vi "niDTS WLAN INSTR TX Fetch DSSS Results.vi"(8 "error in (no error)":errorcluster, 10 "ActiveResultsSpace":u8=1, 11 "niDTS WLAN INSTR TX in":refnum<class "niDTS WLAN INSTR TX.lvclass">) -> (0 "error out":errorcluster, 2 "DSSS Results":T1 {"OBW"."Stop Frequency (Hz)" format="%#_4p"; "OBW"."Start Frequency (Hz)" format="%#_4p"; "OBW"."OBW (Hz)" format="%#_4p"}, 3 "niDTS WLAN INSTR TX out":refnum<class "niDTS WLAN INSTR TX.lvclass">)   [LabVIEW 2015, in "niDTS WLAN.lvlib" / "niDTS WLAN INSTR TX.lvclass"]
uses:
  niDTS WLAN INSTR TX.lvclass
  Tests/Tx Test/Includes/niDTS WLAN Tx Test INC DSSS Results.ctl
  Tests/Tx Test/Includes/niDTS WLAN Tx Test INC DSSS MOD EVM Results.ctl
  Tests/DSSS Tx Test/Includes/Results/niDTS WLAN DSSS Tx RES EVM ALL.ctl
  Tests/DSSS Tx Test/Includes/Results/niDTS WLAN DSSS Tx RES EVM RMS.ctl
  Tests/Tx Test/Includes/niDTS WLAN Tx Test INC TXP Results.ctl
  Tests/Tx Test/Includes/niDTS WLAN Tx Test INC TXP Result SINGLE.ctl
  Tests/Tx Test/Includes/niDTS WLAN Tx Test INC OBW Results.ctl
  Results/niDTS WLAN INSTR TX INC SEM Results.ctl
  Results/niDTS WLAN INSTR TX INC SEM FSEGemts Results.ctl
  Tests/Tx Test/Includes/Results/niDTS Tx RES INC SEM FSEGemts.ctl
  Results/niDTS WLAN INSTR TX INC SEM MARGin Results.ctl
  Tests/Tx Test/Includes/Results/niDTS Tx RES INC SEM Margin.ctl
  Tests/Tx Test/Includes/niDTS WLAN Tx Test INC DSSS MOD Impairments Results.ctl
  Tests/DSSS Tx Test/Includes/Results/niDTS WLAN DSSS Tx Impairmentsctl.ctl
  Tests/DSSS Tx Test/Includes/Results/niDTS WLAN DSSS Tx PowerRamp.ctl
  niDTS WLAN.lvlib
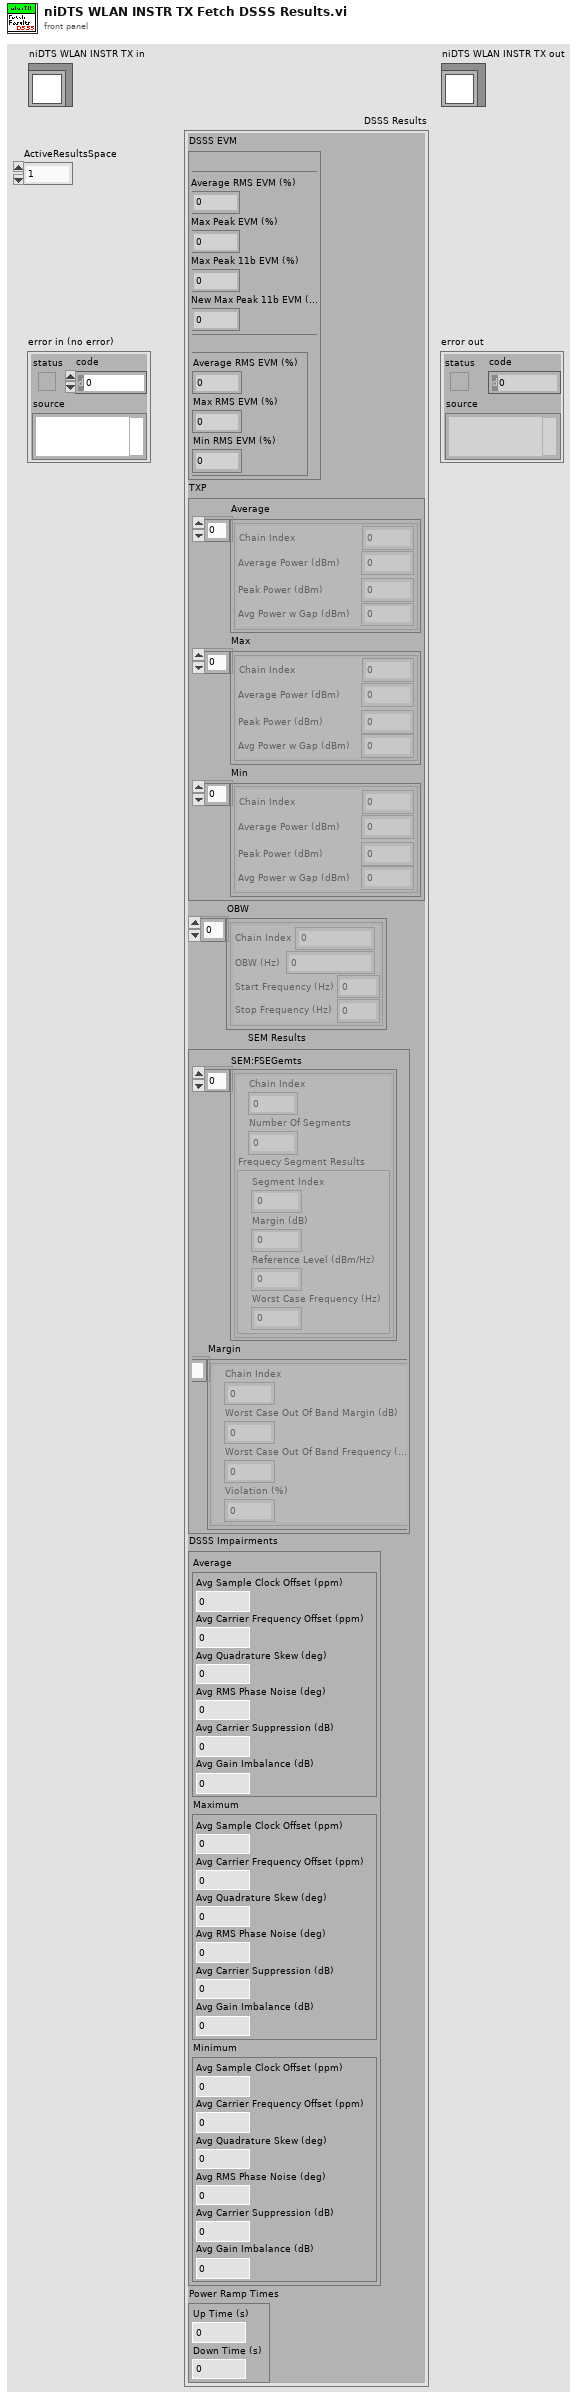
[diagram p1: front panel]
types:
  T1 = typedef "niDTS WLAN.lvlib/niDTS WLAN Tx Test INC DSSS Results.ctl" = cluster{"DSSS EVM":T2, "TXP":T5, "OBW":T7[], "SEM Results":T8, "DSSS Impairments":T13, "Power Ramp Times":T15}
  T2 = typedef "niDTS WLAN.lvlib/niDTS WLAN Tx Test INC DSSS MOD EVM Results.ctl" = cluster{"All":T3, "RMS":T4}
  T3 = typedef "niDTS WLAN.lvlib/niDTS WLAN DSSS Tx RES EVM ALL.ctl" = cluster{"Average RMS EVM (%)":dbl, "Max Peak EVM (%)":dbl, "Max Peak 11b EVM (%)":dbl, "New Max Peak 11b EVM (%)":dbl}
  T4 = typedef "niDTS WLAN.lvlib/niDTS WLAN DSSS Tx RES EVM RMS.ctl" = cluster{"Average RMS EVM (%)":dbl, "Max RMS EVM (%)":dbl, "Min RMS EVM (%)":dbl}
  T5 = typedef "niDTS WLAN.lvlib/niDTS WLAN Tx Test INC TXP Results.ctl" = cluster{"Average":T6[], "Max":T6[], "Min":T6[]}
  T6 = typedef "niDTS WLAN.lvlib/niDTS WLAN Tx Test INC TXP Result SINGLE.ctl" = cluster{"Chain Index":dbl, "Average Power (dBm)":dbl, "Peak Power (dBm)":dbl, "Avg Power w Gap (dBm)":dbl}
  T7 = typedef "niDTS WLAN.lvlib/niDTS WLAN Tx Test INC OBW Results.ctl" = cluster{"Chain Index":dbl, "OBW (Hz)":dbl, "Start Frequency (Hz)":dbl, "Stop Frequency (Hz)":dbl}
  T8 = typedef "niDTS WLAN.lvlib/niDTS WLAN INSTR TX.lvclass/niDTS WLAN INSTR TX INC SEM Results.ctl" = cluster{"SEM:FSEGemts":T9, "Margin":T11}
  T9 = typedef "niDTS WLAN.lvlib/niDTS WLAN INSTR TX.lvclass/niDTS WLAN INSTR TX INC SEM FSEGemts Results.ctl" = T10[]
  T10 = typedef "niDTS WLAN.lvlib/niDTS Tx RES INC SEM FSEGemts.ctl" = cluster{"Chain Index":i32, "Number Of Segments":i32, "Frequecy Segment Results":cluster{"Segment Index":i32, "Margin (dB)":dbl, "Reference Level (dBm/Hz)":dbl, "Worst Case Frequency (Hz)":dbl}}
  T11 = typedef "niDTS WLAN.lvlib/niDTS WLAN INSTR TX.lvclass/niDTS WLAN INSTR TX INC SEM MARGin Results.ctl" = T12[]
  T12 = typedef "niDTS WLAN.lvlib/niDTS Tx RES INC SEM Margin.ctl" = cluster{"Chain Index":i32, "Worst Case Out Of Band Margin (dB)":dbl, "Worst Case Out Of Band Frequency (Hz)":dbl, "Violation (%)":dbl}
  T13 = typedef "niDTS WLAN.lvlib/niDTS WLAN Tx Test INC DSSS MOD Impairments Results.ctl" = cluster{"Average":T14, "Maximum":T14, "Minimum":T14}
  T14 = typedef "niDTS WLAN.lvlib/niDTS WLAN DSSS Tx Impairmentsctl.ctl" = cluster{"Avg Sample Clock Offset (ppm)":dbl, "Avg Carrier Frequency Offset (ppm)":dbl, "Avg Quadrature Skew (deg)":dbl, "Avg RMS Phase Noise (deg)":dbl, "Avg Carrier Suppression (dB)":dbl, "Avg Gain Imbalance (dB)":dbl}
  T15 = typedef "niDTS WLAN.lvlib/niDTS WLAN DSSS Tx PowerRamp.ctl" = cluster{"Up Time (s)":dbl, "Down Time (s)":dbl}
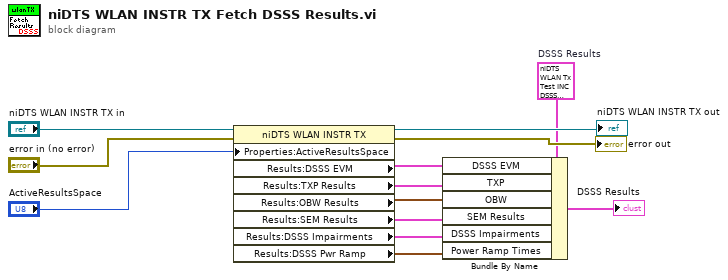
[diagram p0: block diagram]
diagram:
  w8 = T1 {"DSSS EVM"={"All"={"Average RMS EVM (%)"=0.0, "Max Peak EVM (%)"=0.0, "Max Peak 11b EVM (%)"=0.0, "New Max Peak 11b EVM (%)"=0.0}, "RMS"={"Average RMS EVM (%)"=0.0, "Max RMS EVM (%)"=0.0, "Min RMS EVM (%)"=0.0}}, "TXP"={"Average"=[], "Max"=[], "Min"=[]}, "OBW"=[], "SEM Results"={"SEM:FSEGemts"=[], "Margin"=[]}, "DSSS Impairments"={"Average"={"Avg Sample Clock Offset (ppm)"=0.0, "Avg Carrier Frequency Offset (ppm)"=0.0, "Avg Quadrature Skew (deg)"=0.0, "Avg RMS Phase Noise (deg)"=0.0, "Avg Carrier Suppression (dB)"=0.0, "Avg Gain Imbalance (dB)"=0.0}, "Maximum"={"Avg Sample Clock Offset (ppm)"=0.0, "Avg Carrier Frequency Offset (ppm)"=0.0, "Avg Quadrature Skew (deg)"=0.0, "Avg RMS Phase Noise (deg)"=0.0, "Avg Carrier Suppression (dB)"=0.0, "Avg Gain Imbalance (dB)"=0.0}, "Minimum"={"Avg Sample Clock Offset (ppm)"=0.0, "Avg Carrier Frequency Offset (ppm)"=0.0, "Avg Quadrature Skew (deg)"=0.0, "Avg RMS Phase Noise (deg)"=0.0, "Avg Carrier Suppression (dB)"=0.0, "Avg Gain Imbalance (dB)"=0.0}}, "Power Ramp Times"={"Up Time (s)"=0.0, "Down Time (s)"=0.0}}  # DSSS Results
  n1 = property class="niDTS WLAN INSTR TX"(reference="niDTS WLAN INSTR TX in", error in="error in (no error)", "Properties:ActiveResultsSpace"="ActiveResultsSpace") -> (reference out=→"niDTS WLAN INSTR TX out":refnum<class "niDTS WLAN INSTR TX.lvclass">, error out=→"error out":errorcluster, "Results:DSSS EVM"=w7:T2, "Results:TXP Results"=w6:T5, "Results:OBW Results"=w5:T7[], "Results:SEM Results"=w4:T8, "Results:DSSS Impairments"=w3:T13, "Results:DSSS Pwr Ramp"=w2:T15)
  n2 = Bundle By Name(cluster=w8, "DSSS EVM"=w7, "TXP"=w6, "OBW"=w5, "SEM Results"=w4, "DSSS Impairments"=w3, "Power Ramp Times"=w2) -> (→"DSSS Results":T1)
